vi "Finalize Settings 1.0.vi"(8 "error in (no error)":errorcluster, 11 "configuration 1.0":T1={"name"="Group", "direction"=enum."Tx", "cycle timing"={"priority"=100, "decimation"=1, "offset"=0}, "timeout behavior"=enum."Increment Late Count", "enable conversion"=FALSE}) -> (0 "error out":errorcluster, 2 "settings version":T2, 3 "settings":cluster{"key":string, "value":string}[](array[cluster]))   [LabVIEW 2019, in "DSF Core.lvlib" / "Group Configuration.lvclass"]
uses:
  Group Configuration.lvclass
  Typedefs/DSF Version Info.ctl
  DSF Core.lvlib
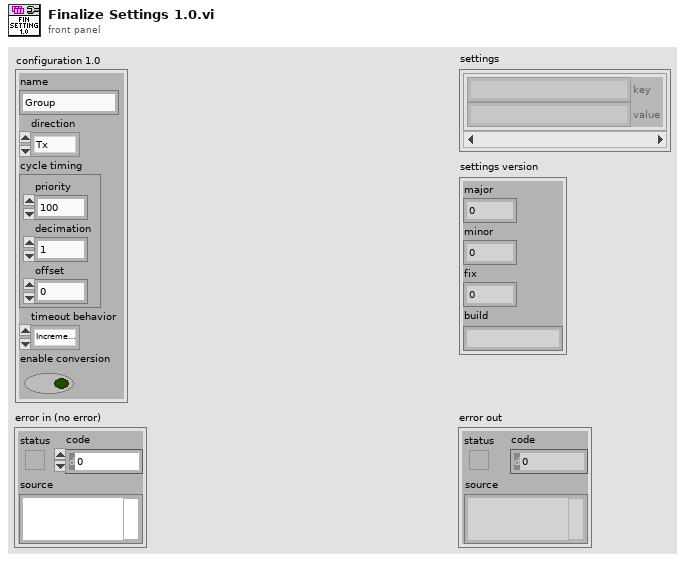
[diagram p1: front panel]
types:
  T1 = cluster{"name":string, "direction":enum8{"Tx", "Rx"}, "cycle timing":cluster{"priority":u64, "decimation":u64, "offset":u64}, "timeout behavior":enum8{"Increment Late Count", "Throw Error"}, "enable conversion":bool}
  T2 = typedef "DSF Core.lvlib/DSF Version Info.ctl" = cluster{"major":u32, "minor":u32, "fix":u32, "build":string}
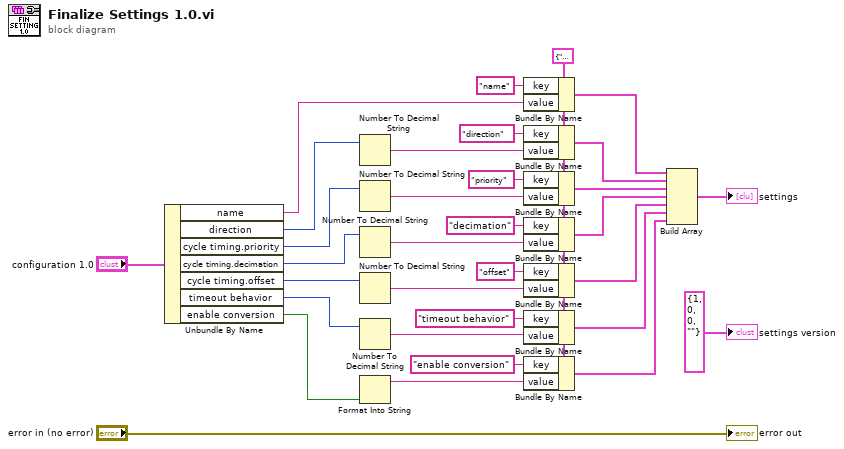
[diagram p0: block diagram]
diagram:
  w5 = cluster{"key":string, "value":string} {"key"="", "value"=""} ("setting")
  n1 = Unbundle By Name("configuration 1.0") -> ("name"=w24:string, "direction"=w15:enum8{"Tx", "Rx"}, "cycle timing.priority"=w20:u64, "cycle timing.decimation"=w19:u64, "cycle timing.offset"=w18:u64, "timeout behavior"=w11:enum8{"Increment Late Count", "Throw Error"}, "enable conversion"=w4:bool)
  n2 = Number To Decimal String(number=w15) -> (decimal integer string=w14:string)  [unwired: 1 in]
  n3 = Number To Decimal String(number=w20) -> (decimal integer string=w23:string)  [unwired: 1 in]
  n4 = Number To Decimal String(number=w19) -> (decimal integer string=w22:string)  [unwired: 1 in]
  n5 = Number To Decimal String(number=w18) -> (decimal integer string=w21:string)  [unwired: 1 in]
  n6 = Number To Decimal String(number=w11) -> (decimal integer string=w9:string)  [unwired: 1 in]
  n7 = Format Into String(w4) -> (resulting string=w3:string)  [unwired: 3 in, 1 out]
  n8 = Bundle By Name(cluster=w5, "key"="name", "value"=w24) -> (w32:cluster{"key":string, "value":string})
  n9 = Bundle By Name(cluster=w5, "key"="direction", "value"=w14) -> (w1:cluster{"key":string, "value":string})
  n10 = Bundle By Name(cluster=w5, "key"="priority", "value"=w23) -> (w31:cluster{"key":string, "value":string})
  n11 = Bundle By Name(cluster=w5, "key"="decimation", "value"=w22) -> (w30:cluster{"key":string, "value":string})
  n12 = Bundle By Name(cluster=w5, "key"="offset", "value"=w21) -> (w17:cluster{"key":string, "value":string})
  n13 = Bundle By Name(cluster=w5, "key"="timeout behavior", "value"=w9) -> (w8:cluster{"key":string, "value":string})
  n14 = Bundle By Name(cluster=w5, "key"="enable conversion", "value"=w3) -> (w2:cluster{"key":string, "value":string})
  n15 = Build Array(w32, w1, w31, w30, w17, w8, w2) -> (→"settings":cluster{"key":string, "value":string}[])
  "error out" <- "error in (no error)"
  "settings version" <- T2 {"major"=1, "minor"=0, "fix"=0, "build"=""} ("settings version")
